vi "CollectData.vi"(4 "Error In":errorcluster, 5 "SimErr":bool=TRUE) -> (0 "Error Out":errorcluster, 2 "Data":dbl[](array[numeric]))   [LabVIEW 2020]
doc: "Dummy VI which simulate collecting some data from some device."
panel:
  out "Progress bar":i32(slide) scale=0.0..100.0
  out "Chart":dbl(graph)
  # "Poczekaj ! Zbieram dane !"
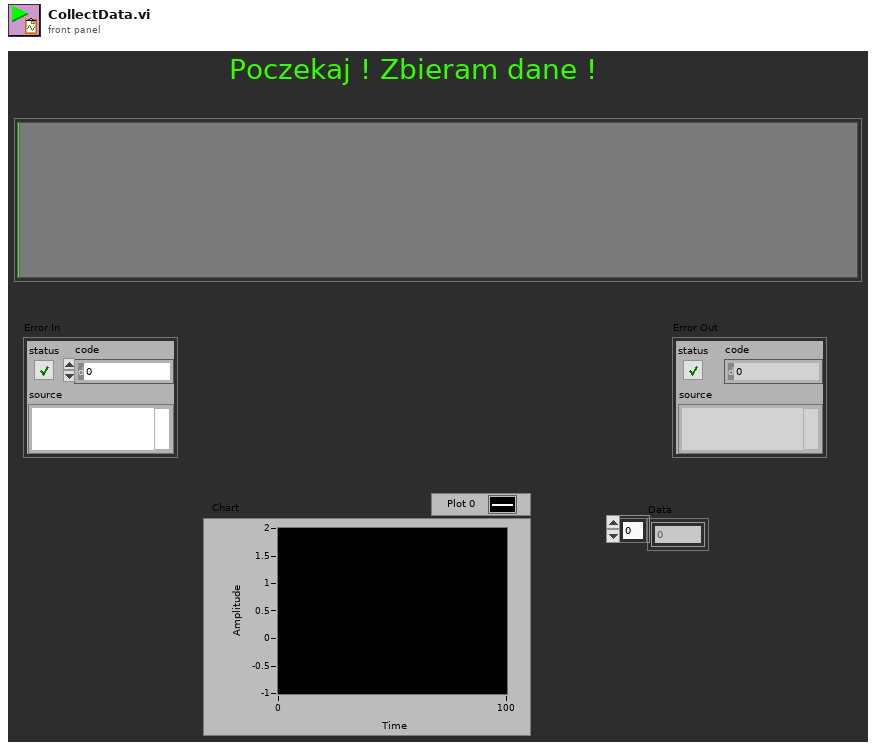
[diagram p1: front panel]
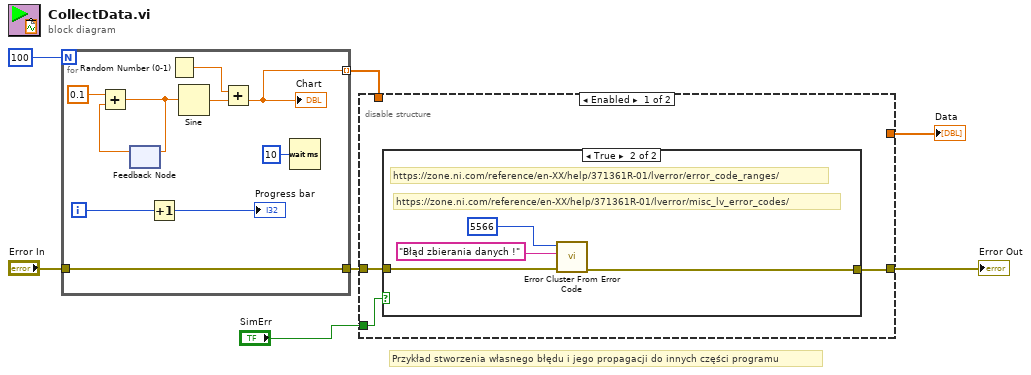
[diagram p0: block diagram]
diagram:
  # "Przykład stworzenia własnego błędu i jego propagacji do innych części programu"
  n1 = for {
    N: 100 -> [_]
    tunnel: [w9] -> w2 mode=indexing
    tunnel: "Error In" -> [w10]
    tunnel: [w10] -> w5
    i -> [w13]
    n2 = feedback #1() -> (w15:dbl)  [unwired: 1 in]
    n3 = Add(x=0.1, y=w15) -> (x+y=w17:dbl)
    n4 = feedback-in #1(w17) -> ()
    n5 = Increment(x=w13) -> (x+1=→"Progress bar":i32)
    n6 = Random Number (0-1)() -> (number: 0 to 1=w8:dbl)
    n7 = Sine(x=w17) -> (sin(x)=w14:dbl)
    n8 = Add(x=w8, y=w14) -> (x+y=w9:dbl)
    "Chart" <- w9
    n9 = Wait (ms)(milliseconds to wait=u32 10) -> ()  [unwired: 1 out]
  }
  n10 = disable-structure shown="Enabled" {
    disable-tunnel: w5 -> [w20 w27]
    disable-tunnel: [w19 w27] -> w4
    disable-tunnel: "SimErr" -> [w18 _]
    disable-tunnel: w2 -> [_ w26]
    disable-tunnel: [_ w26] -> w1
    frame Enabled {
      n11 = case shown="True" w18 {
        tunnel: w20 -> [w21 w25]
        tunnel: [w21 w24] -> w19
        frame False {
        }
        frame True {
          # "https://zone.ni.com/reference/en-XX/help/371361R-01/lverror/misc_lv_error_codes/"
          # "https://zone.ni.com/reference/en-XX/help/371361R-01/lverror/error_code_ranges/"
          n12 = call <vilib>:"Error Cluster From Error Code.vi"("error in (no error)"=w25, "error message (\"\")"="Błąd zbierania danych !" ("error message (\"\")"), "error code (0)"=5566) -> ("error out"=w24:errorcluster)  [unwired: 6 in]
        }
      }
    }
    frame Disabled {
    }
  }
  "Data" <- w1
  "Error Out" <- w4
